vi "GOERTZ END.vi"(2 "L_s(n-2)":dbl[](array[numeric]), 3 "L_s(n-1)":dbl[](array[numeric]), 4 "H_s(n-2)":dbl[](array[numeric]), 5 "H_s(n-1)":dbl[](array[numeric])) -> (0 "L_mag":dbl[](array[numeric]), 1 "H_mag":dbl[](array[numeric]))   [LabVIEW 2020]
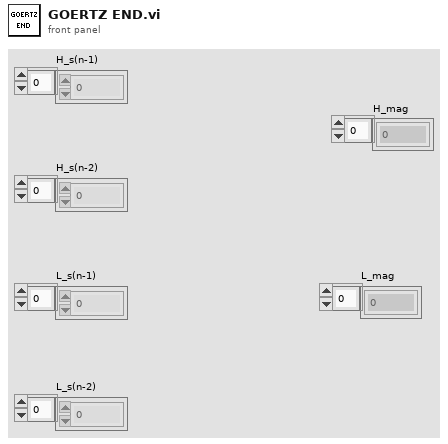
[diagram p1: front panel]
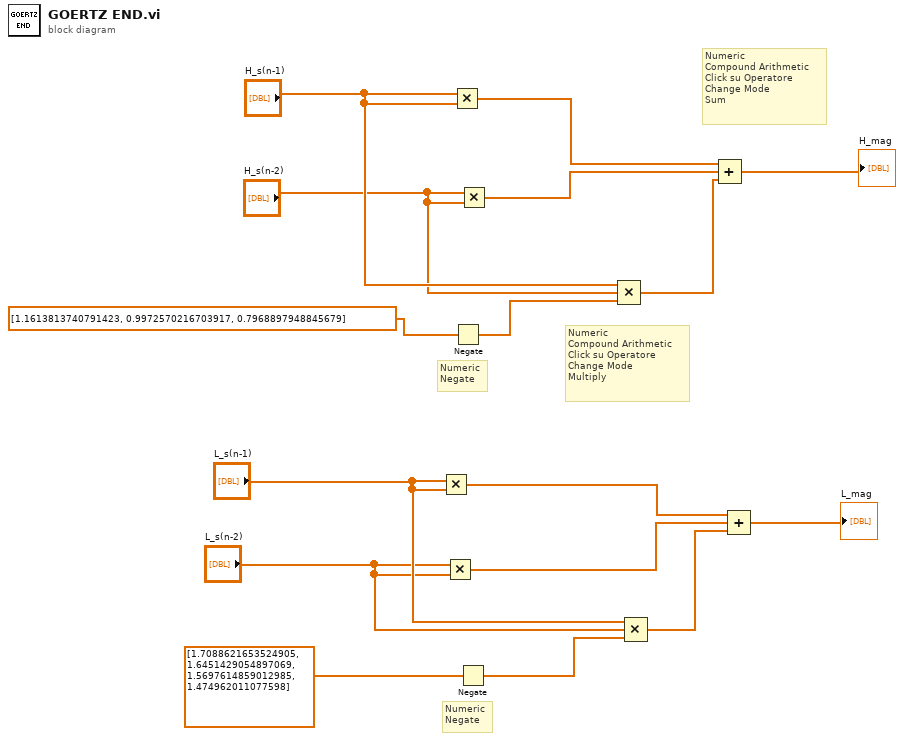
[diagram p0: block diagram]
diagram:
  # "Numeric\nNegate"
  # "Numeric\nNegate"
  # "Numeric\nCompound Arithmetic\nClick su Operatore\nChange Mode\nMultiply"
  # "Numeric\nCompound Arithmetic\nClick su Operatore\nChange Mode\nSum"
  n1 = Multiply(x="L_s(n-1)", y="L_s(n-1)") -> (x*y=w7:dbl[])
  n2 = Multiply(x="L_s(n-2)", y="L_s(n-2)") -> (x*y=w6:dbl[])
  n3 = Multiply(x="H_s(n-1)", y="H_s(n-1)") -> (x*y=w12:dbl[])
  n4 = Negate(x=dbl[] [1.1613813740791423, 0.9972570216703917, 0.7968897948845679] ("2cos(H)")) -> (-x=w13:dbl[])
  n5 = Negate(x=dbl[] [1.7088621653524905, 1.6451429054897069, 1.5697614859012985, 1.474962011077598] ("2cos(L)")) -> (-x=w2:dbl[])
  n6 = Multiply(x="H_s(n-2)", y="H_s(n-2)") -> (x*y=w11:dbl[])
  n7 = Compound Arithmetic op=MULTIPLY("H_s(n-1)", "H_s(n-2)", w13) -> (w10:dbl[])
  n8 = Compound Arithmetic op=MULTIPLY("L_s(n-1)", "L_s(n-2)", w2) -> (w5:dbl[])
  n9 = Compound Arithmetic op=ADD(w12, w11, w10) -> (→"H_mag":dbl[])
  n10 = Compound Arithmetic op=ADD(w7, w6, w5) -> (→"L_mag":dbl[])
